vi "Pre Core.vi"(8 "error in (no error)":errorcluster, 11 "Simple Actor in":refnum<class "Simple Actor.lvclass">) -> (0 "error out":errorcluster, 3 "Simple Actor out":refnum<class "Simple Actor.lvclass">)   [LabVIEW 2020, in "Simple Actor.lvlib" / "Simple Actor.lvclass"]
uses:
  Simple Actor.lvclass
  Actor Msg/Actor Msg.lvclass
  Simple Actor.lvclass/Simple Actor.ctl
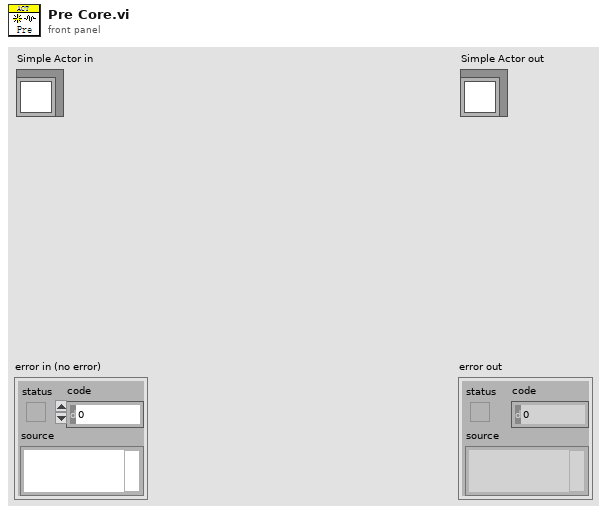
[diagram p1: front panel]
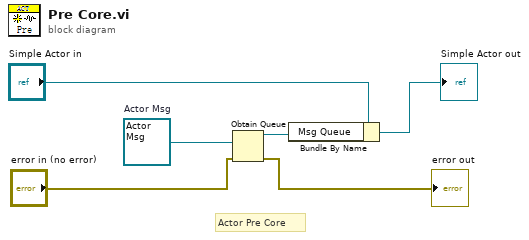
[diagram p0: block diagram]
diagram:
  w4 = refnum<class "Actor Msg.lvclass"> refnum  # Actor Msg
  # "Actor Pre Core"
  n1 = Obtain Queue(element data type=w4, error in (no error)="error in (no error)") -> (queue out=w3:refnum<queue>, error out=→"error out":errorcluster)  [unwired: 3 in, 1 out]
  n2 = Bundle By Name(cluster="Simple Actor in", "Msg Queue"=w3) -> (→"Simple Actor out":refnum<class "Simple Actor.lvclass">)
